vi "fpga_get_scan_ini.vi"(6 "Read Target":bool=TRUE, 8 "initial positions (manual)":T2, 9 "index offset (manual)":T1, 10 "scan (manual)":bool, 11 "scanning":bool) -> (0 "initial positions":T2, 1 "index offfset":T1, 3 "new scan?":bool)   [LabVIEW 2021]
doc: "Get an initial condition for the scan.\n\nDuring the scan, index offset and initial position are stored in this vi. When the scan is turned off, we try to get a new scanning initial condition. When the scan (manual) is true, then we use a new initial condition with \"index offset (manual)\" and \"initial positions (manual)\", otherwise, we try to get these parameters from the DMA."
uses:
  fpga_dtype_index.ctl
  fpga_dtype_sgl_8ch.ctl
  <vilib>/rvi/interface/RandomDataEmulation/niFpgaRandomDataHandleErrors.vi
  <vilib>/rvi/interface/RandomDataEmulation/nirviRandomDataMultiElementFPGAFIFO.vi
  <instcachedir>/0/nirviRandomDataMultiElementFPGAFIFO_3E9965BA1FAD4E7B8DABA31768A09B1F.lvgen/nirviRandomDataMultiElementFPGAFIFO_3E9965BA1FAD4E7B8DABA31768A09B1F_001.vi
  <vilib>/rvi/DataTransferAndStorage/Container/Common/niFpgaContainerExecOnDevCompGetState.vi
  <vilib>/rvi/Emulation/niFpgaEmulationIsFPGAContextNoSignature.vi
  <vilib>/rvi/Emulation/niFpgaSctlEmulationGetInTimedLoop.vi
  <vilib>/rvi/errors/niFpgaSetErrorForExecOnDevCompSimple.vi
  <vilib>/rvi/eio/common/nirviEmuReportErrorAndStop.vi
  <vilib>/rvi/DataTransferAndStorage/Container/Common/niFpgaContainerGetUniqueNameForEmu.vi
  <vilib>/rvi/FIFO/Fifo_Resource/nirvififoEmulationSetSize.vi
  <vilib>/rvi/FIFO/Fifo_Resource/nirviFifoEmulationQueueMgr.vi
  <instcachedir>/0/nirviFifoEmulationQueueMgr_E5CAEC123FF24DC58D834DCA3CDAA9B5.lvgen/nirviFifoEmulationQueueMgr_E5CAEC123FF24DC58D834DCA3CDAA9B5_000.vi
  <vilib>/rvi/FIFO/Fifo_Resource/nirvififoEmulationDetermineInputValidOut.vi
  <vilib>/rvi/FIFO/Fifo_Resource/nirvififoEmulationCreateLock.vi
  <vilib>/rvi/Emulation/niFpgaProcessEmulError.vi
  <vilib>/rvi/FIFO/Fifo_Resource/nirvififoEmulationObtainLock.vi
  <vilib>/rvi/FIFO/Fifo_Resource/nirvififoEmulationReleaseLock.vi
  <vilib>/rvi/occurrence/nirviWaitOnOccurrenceBase.vi
  <vilib>/rvi/errors/nirviReportUnexpectedCaseInternalError.vi
  <vilib>/rvi/errors/nirviReportUnexpectedCaseInternalError (U32).vi
  <vilib>/Utility/error.llb/Clear Errors.vi
  <vilib>/rvi/interface/RandomDataEmulation/nirviRandomDataAcquireLock.vi
  <vilib>/rvi/interface/RandomDataEmulation/nirviRandomDataQueueStore.vi
  <vilib>/rvi/interface/RandomDataEmulation/nirviRandomDataReleaseLock.vi
  <vilib>/rvi/interface/RandomDataEmulation/nirviFPGAContextMergeError.vi
  <vilib>/rvi/interface/RandomDataEmulation/nirviRandomDataCheckExitLoopConditions.vi
  <vilib>/express/rvi/timingcommon/nirviCommon.vi
  <vilib>/rvi/DataTransferAndStorage/Container/XNode/niFpgaContainer.xnode
  <vilib>/rvi/interface/RandomDataEmulation/nirviRandomDataFpgaReadWriteTemplate.vi
  <vilib>/rvi/interface/RandomDataEmulation/nirviRandomDataFpgaMultiElementTemplate.vi
  <vilib>/rvi/FIFO/Fifo_Resource/niFpgaFifoEmulationRefIn.vi
  <vilib>/rvi/FIFO/Fifo_Resource/niFpgaFifoEmulationRefInMultiElement.vi
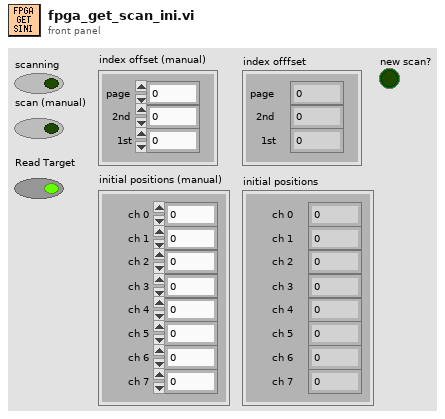
[diagram p1: front panel]
types:
  T1 = typedef "fpga_dtype_index.ctl" = cluster{"page":i16, "2nd":i16, "1st":i16}
  T2 = typedef "fpga_dtype_sgl_8ch.ctl" = cluster{"ch 0":sgl, "ch 1":sgl, "ch 2":sgl, "ch 3":sgl, "ch 4":sgl, "ch 5":sgl, "ch 6":sgl, "ch 7":sgl}
  T3 = cluster{"Element[0]":sgl, "Element[1]":sgl, "Element[2]":sgl, "Element[3]":sgl, "Element[4]":sgl, "Element[5]":sgl, "Element[6]":sgl, "Element[7]":sgl}
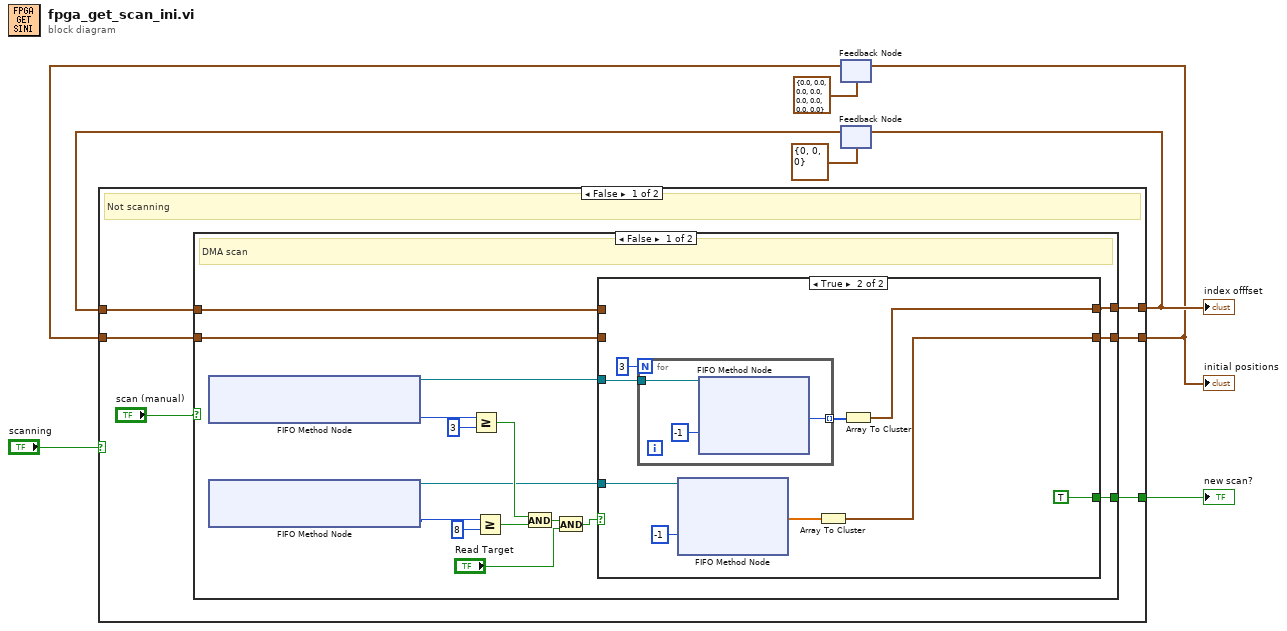
[diagram p0: block diagram]
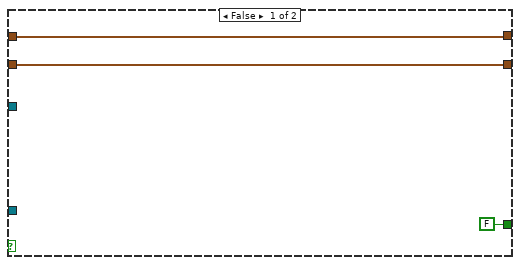
[diagram p2: hidden frame]
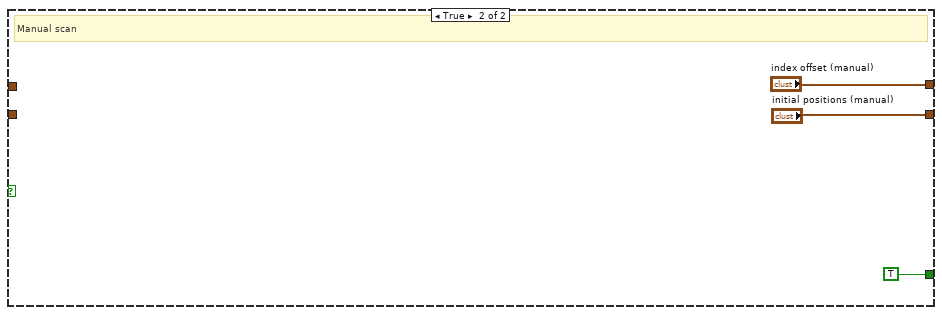
[diagram p3: hidden frame]
diagram:
  n1 = feedback #1(T2 {"ch 0"=0.0, "ch 1"=0.0, "ch 2"=0.0, "ch 3"=0.0, "ch 4"=0.0, "ch 5"=0.0, "ch 6"=0.0, "ch 7"=0.0} ("initial positions")) -> (w5:T2)
  n2 = feedback #2(T1 {"page"=0, "2nd"=0, "1st"=0} ("index offfset")) -> (w6:T1)
  n3 = case shown="False" "scanning" {
    tunnel: w6 -> [w14 w50]
    tunnel: w5 -> [w13 w49]
    tunnel: [w12 w50] -> w4
    tunnel: [w11 w49] -> w2
    tunnel: [w10 _] -> w1
    frame False {
      # "Not scanning"
      n4 = case shown="False" "scan (manual)" {
        tunnel: w14 -> [w22 _]
        tunnel: w13 -> [w21 _]
        tunnel: [w20 "index offset (manual)"] -> w12
        tunnel: [w19 "initial positions (manual)"] -> w11
        tunnel: [w18 TRUE] -> w10
        frame False {
          # "DMA scan"
          n5 = xnode ("FIFO Method Node")() -> ("Number of Elements to Read"=w30:u32, "FIFO Out"=w23:refnum<k21>)  [unwired: 1 in]
          n6 = xnode ("FIFO Method Node")() -> ("Number of Elements to Read"=w29:u32, "FIFO Out"=w24:refnum<k21>)  [unwired: 1 in]
          n7 = Greater Or Equal?(x=w30, y=u32 3) -> (x >= y?=w26:bool)
          n8 = Greater Or Equal?(x=w29, y=u32 8) -> (x >= y?=w25:bool)
          n9 = And(x=w26, y=w25) -> (x .and. y?=w17:bool)
          n10 = And(x=w17, y="Read Target") -> (x .and. y?=w15:bool)
          n11 = case shown="True" w15 {
            tunnel: w24 -> [_ w41]
            tunnel: w23 -> [_ w42]
            tunnel: [w33 w36] -> w20
            tunnel: [w32 w35] -> w19
            tunnel: w22 -> [w33 _]
            tunnel: w21 -> [w32 _]
            tunnel: [FALSE TRUE] -> w18
            frame False {
            }
            frame True {
              n12 = for {
                N: 3 -> [_]
                tunnel: w42 -> [w45]
                tunnel: [w43] -> w37 mode=indexing
                n13 = xnode ("FIFO Method Node")("Timeout"=-1, "FIFO In"=w45) -> ("Element"=w43:i16)  [unwired: 2 out]
              }
              n14 = xnode ("FIFO Method Node")("Timeout"=-1, "FIFO In"=w41) -> ("Element"=w39:sgl[])  [unwired: 2 out]
              n15 = Array To Cluster(array=w39) -> (cluster=w35:T3)
              n16 = Array To Cluster(array=w37) -> (cluster=w36:cluster{"[0]":i16, "[1]":i16, "[2]":i16})
            }
          }
        }
        frame True {
          # "Manual scan"
        }
      }
    }
    frame True {
      # "During the scan, keep index & position data."
    }
  }
  "new scan?" <- w1
  "index offfset" <- w4
  "initial positions" <- w2
  n17 = feedback-in #1(w2) -> ()
  n18 = feedback-in #2(w4) -> ()
